vi "I2C_Decode_Reg_address.vi"(6 "for Ack bit":i32, 8 "Add Points":dbl=10.0, 9 "VDDA":dbl=2.5, 10 "waveform":waveform(dbl), 11 "Index":dbl[](array[numeric])) -> (1 "Reg Address Binary":bool[](array[boolean])=[TRUE, TRUE, TRUE, TRUE, TRUE, FALSE, FALSE, TRUE, TRUE, TRUE, FALSE, TRUE], 2 "Reg Address ACK":bool, 3 "Reg Address":u32=2975 format="%.0x")   [LabVIEW 2019]
panel:
  out "Array 3":dbl[](array[numeric])=[0.03750000000000009, 2.4360937499999995, 0.05249999999999977, -0.05343750000000025, -0.017343750000000213, 2.4328125, 0.20250000000000012, 0.06046875000000007, -0.07593750000000021, 2.4351562499999995, 0.1846874999999999, -0.005156250000000195, 0.0885937499999998, -0.0070312500000002665, 0.5826562500000003, 2.338125, 2.4604687499999995, 0.04921875000000009, 0.05484374999999986, 0.03374999999999995, -0.01171875, 2.3404687499999994, 0.46734374999999995, 0.03937500000000016, 0.06796874999999991, 0.06000000000000005, 0.012187500000000018, 2.40046875, 0.1471874999999998, 0.029999999999999805, 0.03234374999999989, 0.00749999999999984, 0.7846874999999995, 2.4553125, -0.053906250000000266, 0.012187500000000018, -0.07828124999999986, 2.3390625, -0.014531250000000107, -0.08765625000000021, 0.03374999999999995, -0.030468750000000266, 0.08390625000000007, 2.44125, 0.1143749999999999, 0.039843749999999734, -0.020624999999999893, 0.04078124999999977, 0.06421874999999977, 0.07499999999999973, 0.6703124999999996, 2.3864062500000003, 2.32125, 2.39953125]
  out "size(s) 2":i32=14
  out "subarray":dbl[](array[numeric])=[1.0, 0.0, 1.0, 1.0, 1.0, 0.0, 0.0, 1.0, 1.0, 1.0, 1.0, 1.0, 1.0, 1.0]
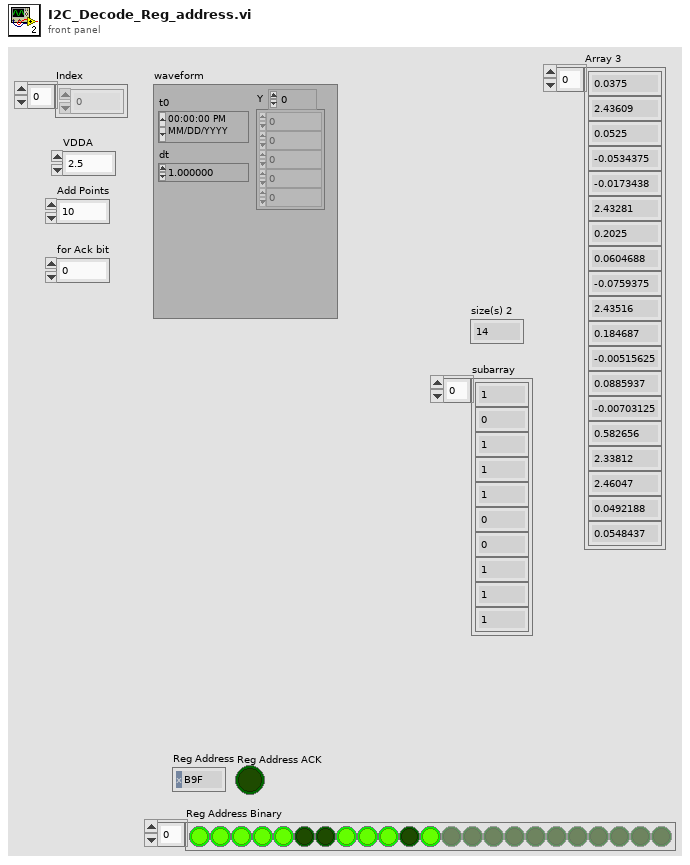
[diagram p1: front panel]
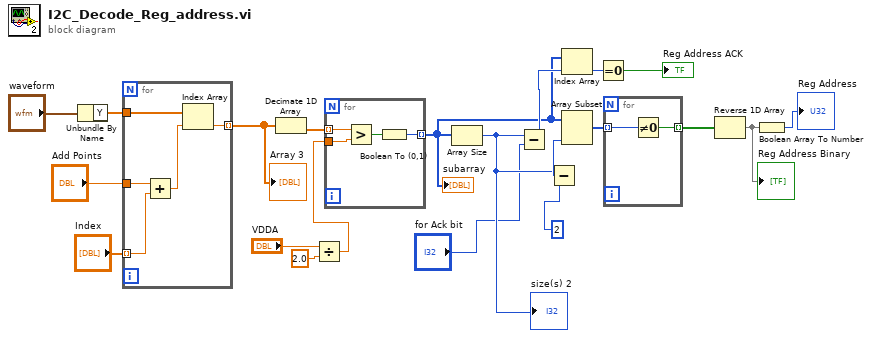
[diagram p0: block diagram]
diagram:
  n1 = Unbundle By Name("waveform") -> ("Y"=w6:dbl[])
  n2 = for {
    tunnel: "Index" -> [w25] mode=indexing
    tunnel: w6 -> [w26]
    tunnel: [w24] -> w21 mode=indexing
    tunnel: "Add Points" -> [w22]
    n3 = Add(x=w22, y=w25) -> (x+y=w23:dbl)
    n4 = Index Array(array=w26, index=w23) -> (element=w24:dbl)
  }
  "Array 3" <- w21
  n5 = Decimate 1D Array(w21) -> (w20:dbl[])  [unwired: 1 out]
  n6 = Divide(x="VDDA", y=2.0) -> (x/y=w18:dbl)
  n7 = for {
    tunnel: w20 -> [w30] mode=indexing
    tunnel: w18 -> [w29]
    tunnel: [w27] -> w7 mode=indexing
    n8 = Greater?(x=w30, y=w29) -> (0:w28:bool)
    n9 = Boolean To (0,1)(Boolean=w28) -> (0, 1=w27:i16)
  }
  "subarray" <- w7
  n10 = Array Size(array=w7) -> (size(s)=w3:i32)
  "size(s) 2" <- w3
  n11 = Subtract(x=w3, y="for Ack bit") -> (x-y=w11:i32)
  n12 = Subtract(x=w3, y=2) -> (x-y=w16:i32)
  n13 = Index Array(array=w7, index=w11) -> (element=w13:i16)
  n14 = Array Subset(array=w7, length=w16) -> (w15:i16[])  [unwired: 1 in]
  n15 = Equal To 0?(x=w13) -> (x = 0?=→"Reg Address ACK":bool)
  n16 = for {
    tunnel: w15 -> [w32] mode=indexing
    tunnel: [w31] -> w9 mode=indexing
    n17 = Not Equal To 0?(x=w32) -> (x != 0?=w31:bool)
  }
  n18 = Reverse 1D Array(array=w9) -> (reversed array=w8:bool[])
  "Reg Address Binary" <- w8
  n19 = Boolean Array To Number(Boolean array=w8) -> (number=→"Reg Address":u32)
